vi "Get Results Name.vi"(8 "error in (no error)":errorcluster, 11 "Pips in":refnum<class "Pips.lvclass">) -> (0 "error out":errorcluster, 2 "Name":string, 3 "Pips out":refnum<class "Pips.lvclass">)   [LabVIEW 2021, in "Bananas.lvlib" / "Pips.lvclass"]
uses:
  Pips.lvclass
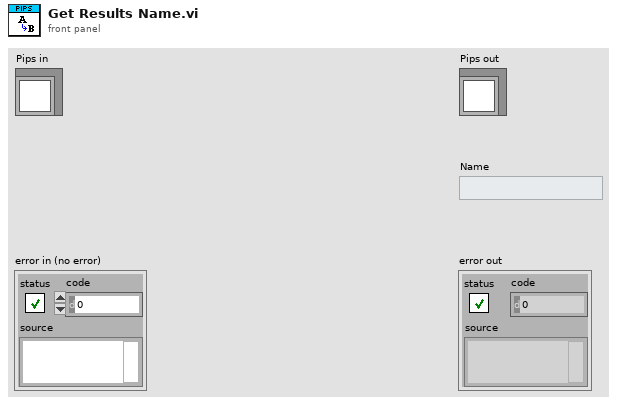
[diagram p1: front panel]
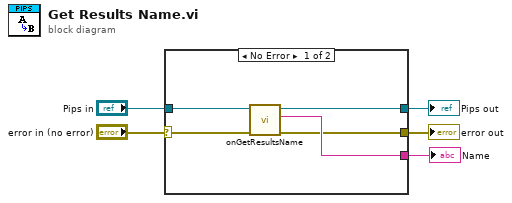
[diagram p0: block diagram]
diagram:
  n1 = case shown="No Error" "error in (no error)" {
    selector: "error in (no error)" -> [w9 w12]
    tunnel: [w6 w12] -> w4
    tunnel: [w8 w11] -> w2
    tunnel: "Pips in" -> [w10 w11]
    tunnel: [w7 _] -> w1
    frame No Error {
      n2 = call-dynamic "onGetResultsName.vi"("error in (no error)"=w9, "Pips in"=w10) -> ("error out"=w6:errorcluster, "Name"=w7:string, "Pips out"=w8:refnum<class "Pips.lvclass">)  [unwired: 7 in]
    }
    frame Error {
    }
  }
  "error out" <- w4
  "Pips out" <- w2
  "Name" <- w1
